vi "hyteresis.vi"(9 "target_temp":i8, 10 "real_temp":dbl, 11 "manual_on":bool) -> (3 "control_signal":bool)   [LabVIEW 2014]
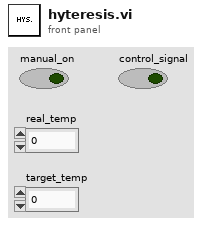
[diagram p1: front panel]
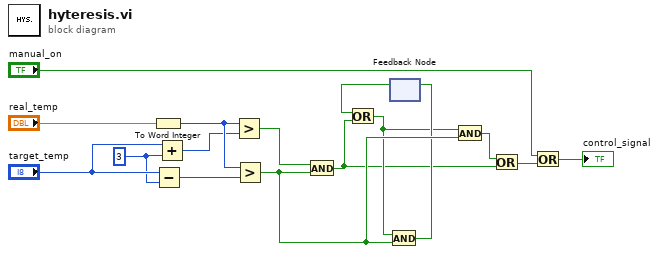
[diagram p0: block diagram]
diagram:
  w4 = 3
  n1 = To Word Integer(number="real_temp") -> (16bit integer=w6:i16)
  n2 = Subtract(x="target_temp", y=w4) -> (x-y=w9:i32)
  n3 = Add(x="target_temp", y=w4) -> (x+y=w3:i32)
  n4 = Greater?(x=w6, y=w3) -> (0:w13:bool)
  n5 = Greater?(x=w6, y=w9) -> (0:w12:bool)
  n6 = And(x=w13, y=w12) -> (x .and. y?=w1:bool)
  n7 = feedback #1() -> (w8:bool)  [unwired: 1 in]
  n8 = Or(x=w8, y=w1) -> (x .or. y?=w2:bool)
  n9 = And(x=w2, y=w12) -> (x .and. y?=w11:bool)
  n10 = feedback-in #1(w11) -> ()
  n11 = And(x=w2, y=w12) -> (x .and. y?=w10:bool)
  n12 = Or(x=w10, y=w1) -> (x .or. y?=w15:bool)
  n13 = Or(x="manual_on", y=w15) -> (x .or. y?=→"control_signal":bool)
